vi "Teleop.vi"(10 "Match Info":T2={"Autonomous Elapsed Seconds"=0.0, "TeleOp Elapsed Seconds"=0.0, "Disabled Elapsed Seconds"=0.0, "Visited Autonomous"=FALSE, "Visited TeleOp"=FALSE, "Visited Disabled"=FALSE, "Autonomous Settings"={"Autonomous Style"=enum."Independent", "VI Refnum"=refnum}}, 11 "Call Context":T1) -> ()   [LabVIEW 2018]
doc: "This VI is called for each TeleOp packet received from the DS where the robot is not disabled. It is often used to read from the joysticks and update I/O or to update setpoints for timed control loops. It should complete and return within 20 milliseconds or it may miss DS packets."
uses:
  <vilib>/Rock Robotics/WPI/DriverStation/WPI_DriverStationMatch Info.ctl
  <vilib>/Rock Robotics/WPI/DriverStation/WPI_DriverStationDerivedRobotMode.ctl
  <vilib>/Rock Robotics/WPI/Utilities/WPI_GetSetVariantRefNum.vi
  <vilib>/Rock Robotics/Network Tables/NT Read Boolean.vi
  <vilib>/Rock Robotics/Network Tables/NT Write Boolean.vi
  <vilib>/Rock Robotics/WPI/Ultrasonic/WPI_UltrasonicRangeUnits.ctl
  <vilib>/Rock Robotics/WPI/Ultrasonic/WPI_SonarSRF04DigitalGetRange.vi
  <vilib>/Rock Robotics/WPI/Ultrasonic/WPI_SonarSRF04DigitalRefNum Registry Get.vi
panel:
  in  "Square Inputs":bool
  in  "Max":dbl=1.0 min=-1.0 max=1.0 step=0.1
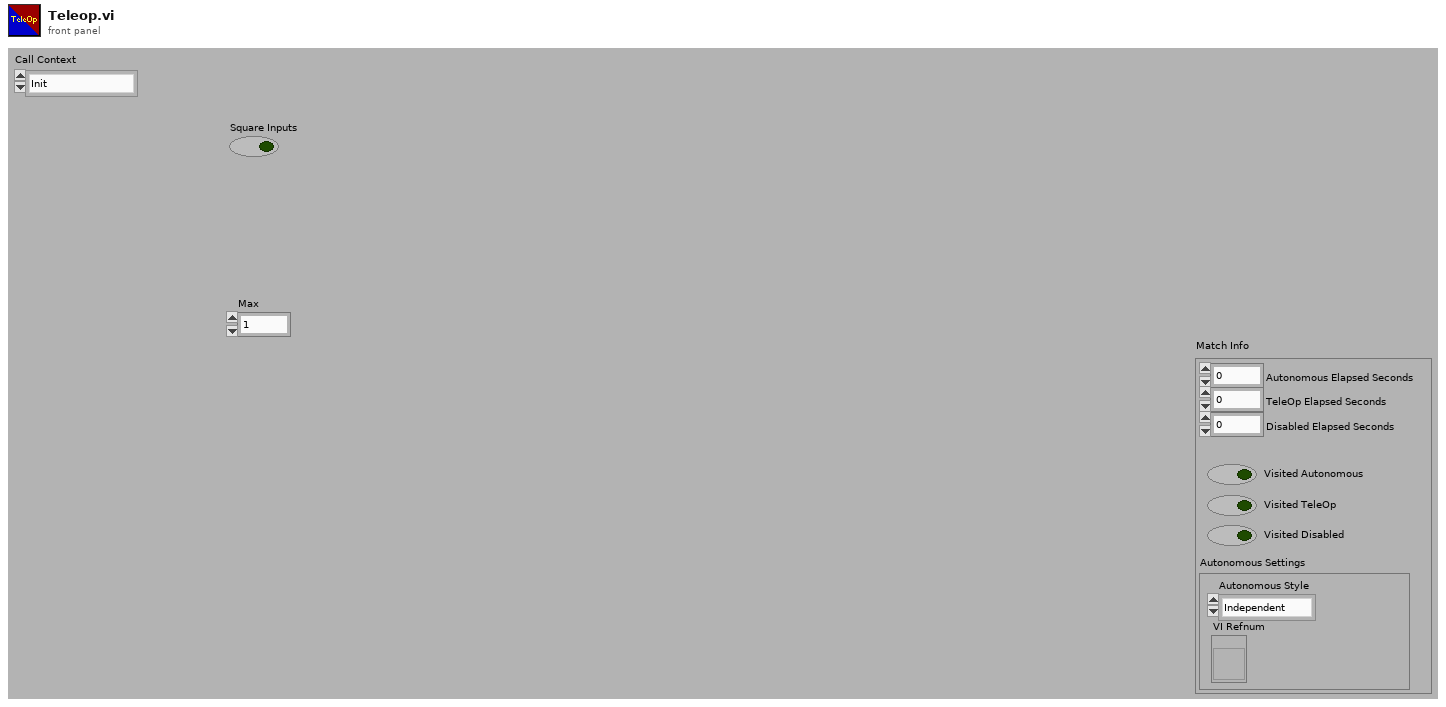
[diagram p1: front panel]
types:
  T1 = typedef "WPI_DriverStationDerivedRobotMode.ctl" = enum16{"Init", "Execute", "Stop"}
  T2 = typedef "WPI_DriverStationMatch Info.ctl" = cluster{"Autonomous Elapsed Seconds":dbl, "TeleOp Elapsed Seconds":dbl, "Disabled Elapsed Seconds":dbl, "Visited Autonomous":bool, "Visited TeleOp":bool, "Visited Disabled":bool, "Autonomous Settings":cluster{"Autonomous Style":enum16{"Iterative", "Independent"}, "VI Refnum":refnum<vi>}}
  T3 = typedef "WPI_UltrasonicRangeUnits.ctl" = enum16{"inches", "mm"}
  T4 = typedef "WPI_UltrasonicDeviceRef.ctl" = cluster{"DevStatus":errorcluster, "Ping Channel":T5, "Echo Channel":T5, "CntIndex":T6}
  T5 = typedef "FPGA_DIOChannel.ctl" = enum8{"DIO 0", "DIO 1", "DIO 2", "DIO 3", "DIO 4", "DIO 5", "DIO 6", "DIO 7", "DIO 8", "DIO 9", "DIO MXP 0", "DIO MXP 1", "DIO MXP 2", "DIO MXP 3", "DIO MXP 4", "DIO MXP 5", "DIO MXP 6", "DIO MXP 7", "DIO MXP 8", "DIO MXP 9", "DIO MXP 10", "DIO MXP 11", "DIO MXP 12", "DIO MXP 13", "DIO MXP 14", "DIO MXP 15", "SPI Port CS1", "SPI Port CS2", "SPI Port CS3", "SPI Port MISO", "SPI Port MOSI", "Invalid"}
  T6 = typedef "FPGA_CounterCtrSystemIndex.ctl" = enum8{"Ctr 0", "Ctr 1", "Ctr 2", "Ctr 3", "Ctr 4", "Ctr 5", "Ctr 6", "Ctr 7", "Invalid"}
  T7 = typedef "WPI_JoystickDevRef.ctl" = cluster{"Device":T8}
  T8 = typedef "WPI_JoystickDeviceEnum.ctl" = enum16{"USB 0", "USB 1", "USB 2", "USB 3", "USB 4", "USB 5"}
  T9 = typedef "WPI_MotorControlDeviceRef.ctl" = cluster{"DeviceStatus":errorcluster, "Type":T10, "PWM":cluster{"PWM Channel":T11, "DeadBand":T12}, "CAN":cluster{"Device Number":u8, "SetOutput VI Ref":variant, "GetOutput VI Ref":variant, "Enable VI Ref":variant, "Disable VI Ref":variant, "Data":variant}, "Invert":bool, "DIO PWM":cluster{"PWM \"Enable\" Channel":T11, "DIOChannel":T5, "PWM Rate":dbl}}
  T10 = typedef "WPI_MotorControlType.ctl" = enum16{"PWM", "CAN", "DIO PWM"}
  T11 = typedef "FPGA_DIOPWMChannel.ctl" = enum8{"PWM 0", "PWM 1", "PWM 2", "PWM 3", "PWM 4", "PWM 5", "PWM 6", "PWM 7", "PWM 8", "PWM 9", "PWM MXP 0", "PWM MXP 1", "PWM MXP 2", "PWM MXP 3", "PWM MXP 4", "PWM MXP 5", "PWM MXP 6", "PWM MXP 7", "PWM MXP 8", "PWM MXP 9", "Invalid"}
  T12 = typedef "WPI_PWMDeadband.ctl" = cluster{"Name":string, "maxPositivePwm":i32, "minPositivePwm":i32, "centerPwm":i32, "maxNegativePwm":i32, "minNegativePwm":i32, "angularRange":u16}
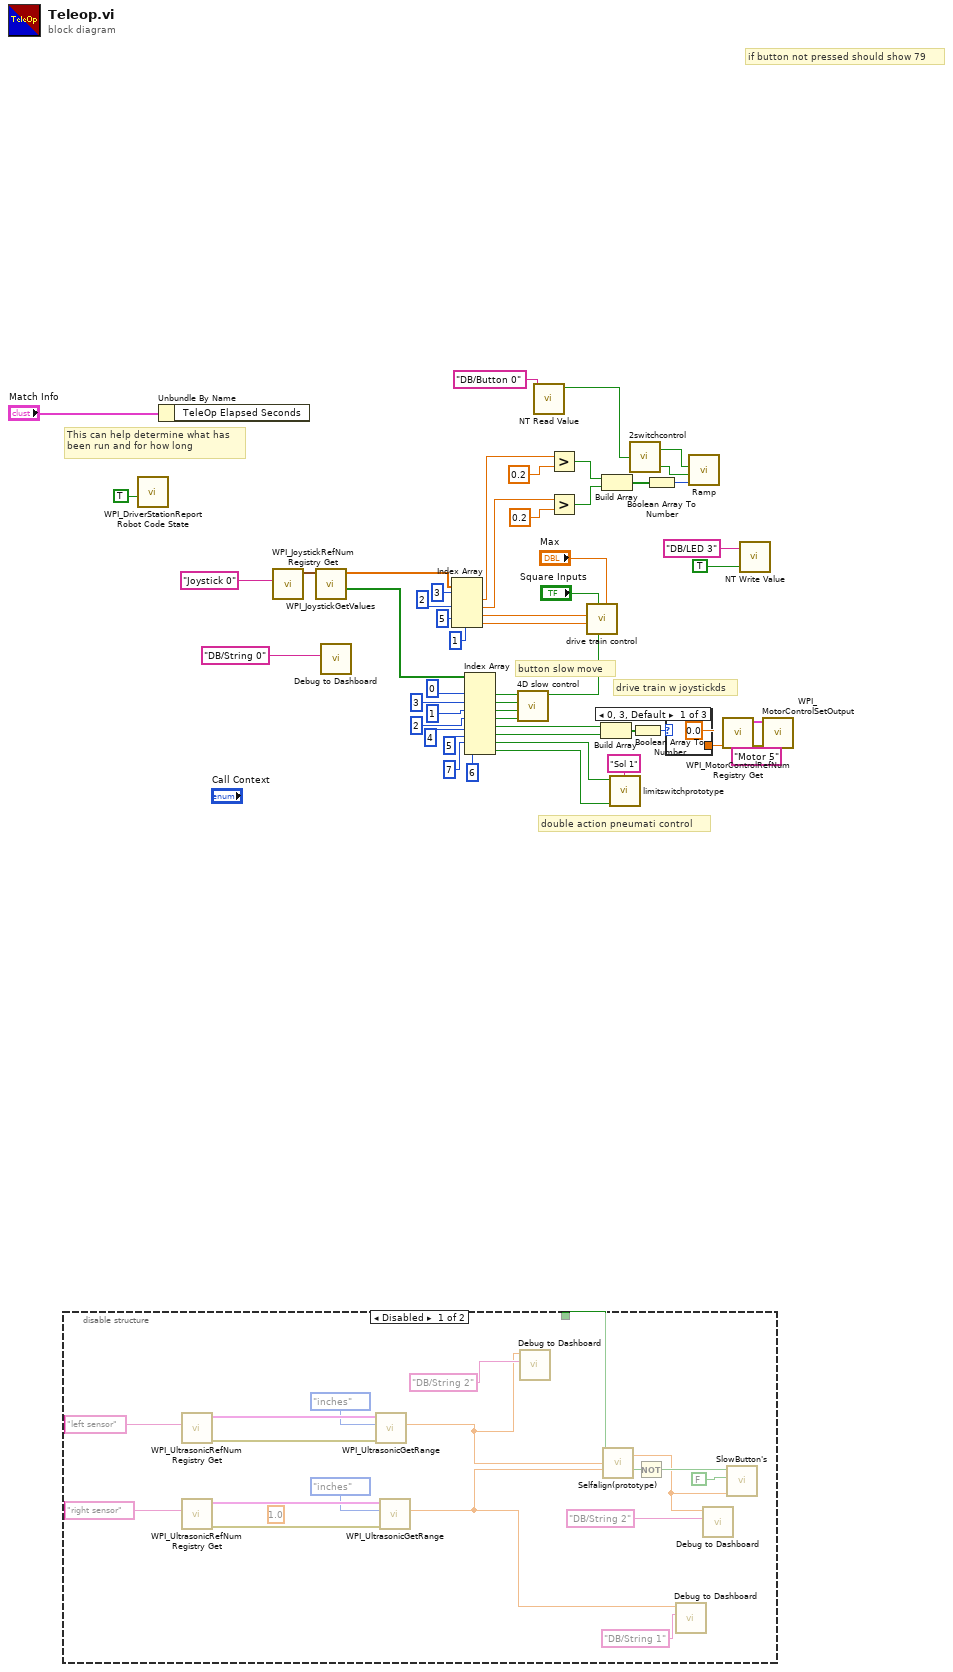
[diagram p0: block diagram]
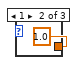
[diagram p3: hidden frame]
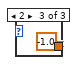
[diagram p4: hidden frame]
diagram:
  # "double action pneumati control"
  # "button slow move"
  # "drive train w joystickds"
  # "if button not pressed should show 79"
  # "This can help determine what has\nbeen run and for how long"
  n1 = disable-structure shown="Disabled" {
    disable-tunnel: _ -> [w60 _]
    frame Disabled {
      (unwired) sgl 1.0 ("ping time (s)")
      n2 = call-poly <vilib>:"WPI_UltrasonicRefNum Registry Get.vi"("refnum name"="left sensor") -> ("error out"=w67:errorcluster, "SonarSRF04DevRef"=w68:T4)  [unwired: 9 in]
      n3 = call-poly <vilib>:"WPI_UltrasonicRefNum Registry Get.vi"("refnum name"="right sensor") -> ("error out"=w70:errorcluster, "SonarSRF04DevRef"=w71:T4)  [unwired: 9 in]
      n4 = call-poly <vilib>:"WPI_UltrasonicGetRange.vi"("error in (no error)"=w67, "ping time (s)"=WPI_UltrasonicRangeUnits."inches" ("Range Units"), "SonarSRF04DevRef"=w68) -> ("Distance"=w56:dbl)  [unwired: 6 in, 2 out]
      n5 = call-poly <vilib>:"WPI_UltrasonicGetRange.vi"("error in (no error)"=w70, "ping time (s)"=WPI_UltrasonicRangeUnits."inches" ("Range Units"), "SonarSRF04DevRef"=w71) -> ("Distance"=w58:dbl)  [unwired: 6 in, 2 out]
      n6 = call "Debug to Dashboard.vi"("NT String Label"="DB/String 2", "input"=w56) -> ()  [unwired: 10 in]
      n7 = call "Selfalign(prototype).vi"("Run"=w60, "Left Distance Output"=w56, "Right Distance Output"=w58) -> ("Motor Speed"=w62:dbl, "The stop that matters"=w64:bool)  [unwired: 11 in]
      n8 = Not(x=w64) -> (.not. x?=w63:bool)
      n9 = call "Debug to Dashboard.vi"("NT String Label"="DB/String 1", "input"=w58) -> ()  [unwired: 10 in]
      n10 = call "Debug to Dashboard.vi"("NT String Label"="DB/String 2", "input"=w62) -> ()  [unwired: 10 in]
      n11 = call "SlowButton's.vi"("Speed"=w62, "Straight"=FALSE, "Run"=w63) -> ()  [unwired: 9 in]
    }
    frame Enabled {
    }
  }
  n12 = call <vilib>:"WPI_DriverStationReport Robot Code State.vi"("TeleOp"=TRUE ("Autonomous")) -> ()  [unwired: 10 in, 1 out]
  n13 = Unbundle By Name("Match Info") -> ()  [unwired: 1 out]
  n14 = call <vilib>:"WPI_JoystickRefNum Registry Get.vi"("refnum name"="Joystick 0") -> ("JoystickDevRef"=w50:T7)  [unwired: 1 in, 9 out]
  n15 = call <vilib>:"WPI_JoystickGetValues.vi"("JoystickDevRef"=w50) -> ("Buttons"=w44:bool[], "Axes"=w47:dbl[])  [unwired: 6 in, 3 out]
  n16 = call "Debug to Dashboard.vi"("NT String Label"="DB/String 0" ("Name")) -> ()  [unwired: 11 in]
  n17 = Index Array(array=w47, index #1=3 ("index"), index #2=2 ("index"), index #3=5, index #4=1) -> (element #1=w27:dbl, element #2=w26:dbl, element #3=w25:dbl, element #4=w24:dbl)
  n18 = Index Array(array=w44, index #1=0, index #2=3, index #3=1, index #4=2, index #5=4, index #6=5 ("index"), index #7=7, index #8=6 ("index")) -> (element #1=w20:bool, element #2=w19:bool, element #3=w18:bool, element #4=w17:bool, element #5=w16:bool, element #6=w15:bool, element #7=w9:bool, element #8=w8:bool)
  n19 = call "4D slow control.vi"("Backward"=w17, "Forward"=w18, "Right"=w19, "Left"=w20) -> ("Running Motor"=w13:bool)  [unwired: 7 in]
  n20 = call-poly <vilib>:"NT Read Value.vi"("Name"="DB/Button 0") -> ("Boolean"=w3:bool)  [unwired: 9 in, 1 out]
  n21 = Greater?(x=w27, y=0.2) -> (0:w11:bool)
  n22 = Greater?(x=w26, y=0.2) -> (0:w12:bool)
  n23 = call "drive train control.vi"("Max"="Max", "take motor input"=w13, "Square Inputs"="Square Inputs", "input 1"=w24, "input 2"=w25) -> ()  [unwired: 7 in]
  n24 = Build Array(w16, w15) -> (w21:bool[])
  n25 = Build Array(w11, w12) -> (w34:bool[])
  n26 = call "limitswitchprototype.vi"("Sol Name"="Sol 1", "Close"=w8, "Open"=w9) -> ()  [unwired: 9 in]
  n27 = call "2switchcontrol.vi"("Overide"=w3) -> ("Switch 1"=w5:bool, "Switch 2"=w4:bool)
  n28 = Boolean Array To Number(Boolean array=w21) -> (number=w30:u32)
  n29 = Boolean Array To Number(Boolean array=w34) -> (number=w6:u32)
  n30 = case shown="0, 3, Default" w30 {
    tunnel: [0.0 1.0 -1.0] -> w38
    frame 0, 3, Default {
    }
    frame 1 {
    }
    frame 2 {
    }
  }
  n31 = call "Ramp.vi"("Control"=w6, "Switch 2"=w4, "Switch 1"=w5) -> ()  [unwired: 9 in]
  n32 = call <vilib>:"WPI_MotorControlRefNum Registry Get.vi"("refnum name"="Motor 5") -> ("error out"=w40:errorcluster, "MotorControlDevRef"=w41:T9)  [unwired: 9 in]
  n33 = call-poly <vilib>:"NT Write Value.vi"("Boolean"=TRUE, "Name"="DB/LED 3") -> ()  [unwired: 9 in, 1 out]
  n34 = call <vilib>:"WPI_MotorControlSetOutput.vi"("error in (no error)"=w40, "Output"=w38, "MotorControlDevRef"=w41) -> ()  [unwired: 6 in, 3 out]
